vi "6514_timeout.vi"() -> ()   [LabVIEW 2015]
panel:
  out "read buffer":string
  out "VISA resource name out":refnum<visa-resource-name>="GPIB0::20::INSTR"
  in  "write buffer":string=":INIT;SENS:DATA?"
  in  "VISA resource name":refnum<visa-resource-name>="GPIB0::20::INSTR"
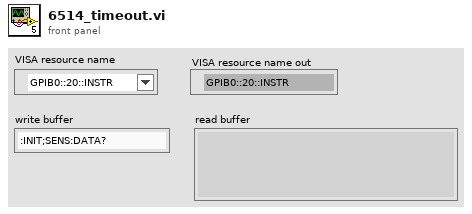
[diagram p1: front panel]
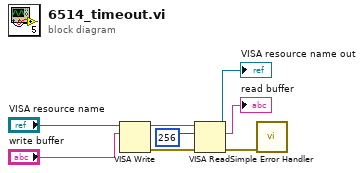
[diagram p0: block diagram]
diagram:
  n1 = VISA Write(VISA resource name="VISA resource name", write buffer="write buffer") -> (VISA resource name out=w6:refnum<visa-resource-name>, error out=w5:errorcluster)  [unwired: 1 in, 1 out]
  n2 = VISA Read(VISA resource name=w6, byte count=u32 256, error in (no error)=w5) -> (VISA resource name out=→"VISA resource name out":refnum<visa-resource-name>, read buffer=→"read buffer":string, error out=w2:errorcluster)  [unwired: 1 out]
  n3 = call <vilib>:"Simple Error Handler.vi"("error in (no error)"=w2) -> ()  [unwired: 4 in, 5 out]
